vi "Compute Max Level.vi"(0 "File in":refnum<class "File.lvclass">, 1 "Filter in":refnum<class "Filter.lvclass">, 5 "Level in":refnum<class "Level.lvclass">, 7 "Fs (Hz)":dbl, 9 "Vmax":dbl, 11 "error in (no error)":errorcluster) -> (4 "File out":refnum<class "File.lvclass">, 6 "Level thru":refnum<class "Level.lvclass">, 10 "Lmax":dbl, 15 "error out":errorcluster)   [LabVIEW 2020, in "File.lvclass"]
uses:
  File.lvclass
  Level/Level.lvclass
  Filter/Filter.lvclass
  Level/Level.lvclass/Level.ctl
  File.lvclass/File.ctl
  aa2963da-88b9-45dc-ab26-109d9a687043.vi
  6b23c93a-1c02-4248-999f-575423126d1e.vi
  439032d3-8d6b-4fc5-a9ed-bfbf51eac51d.vi
  e43c2267-94e9-47ec-9fe9-8526f4fbc379.vi
  Level/Read Units.vi
  Utility VIs/Math VIs/FFT x(t) to dB,Degrees (1D).vi
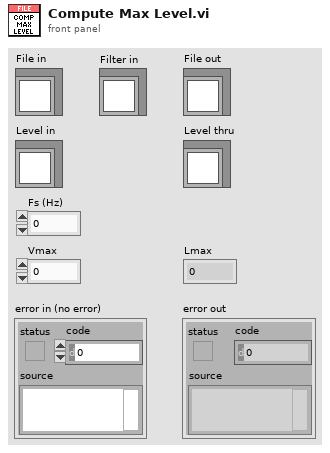
[diagram p1: front panel]
types:
  T1 = typedef "Level.lvclass/LevelUnits.ctl" = enum16{"dB atten", "dB SPL", "dB Vrms", "Volts", "dB mW", "mW", "dB HL", "dB SL"}
  T2 = cluster{"Freq (Hz)":dbl[], "Mag (dB SPL)":dbl[], "Phase (deg)":dbl[]}
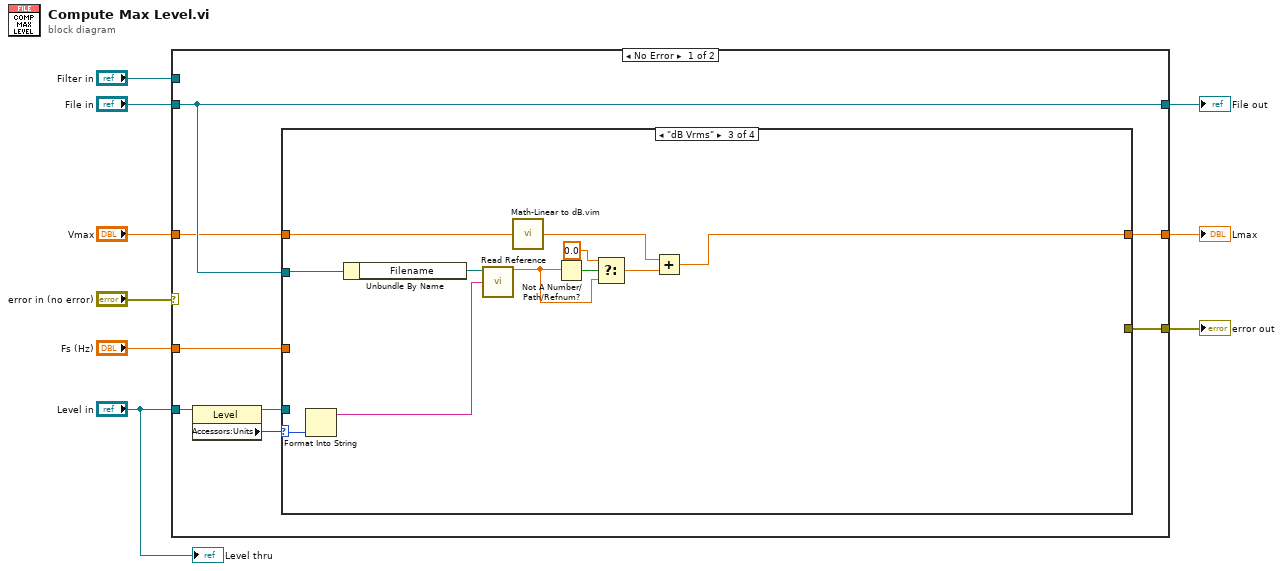
[diagram p0: block diagram]
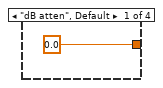
[diagram p2: hidden frame]
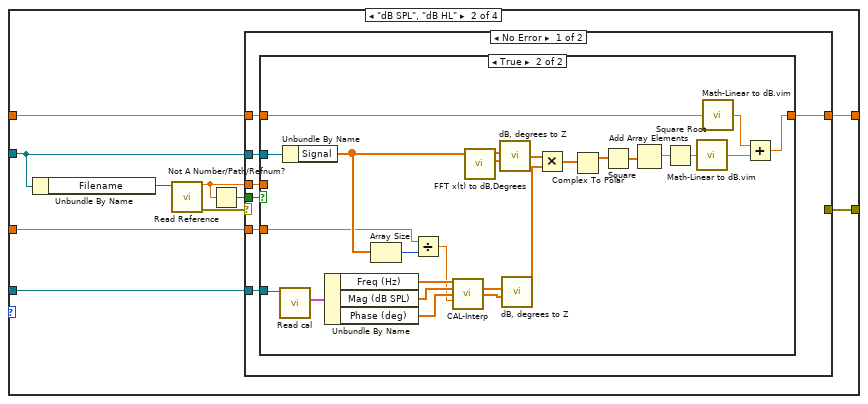
[diagram p3: hidden frame]
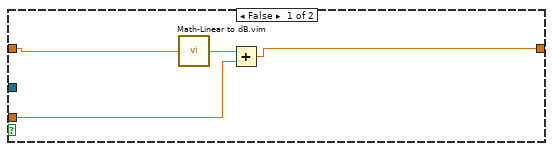
[diagram p4: hidden frame]
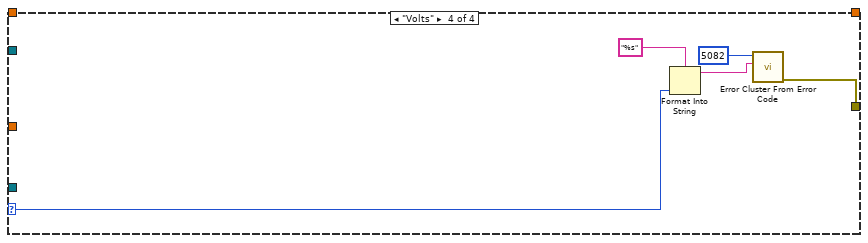
[diagram p6: hidden frame]
diagram:
  n1 = case shown="No Error" "error in (no error)" {
    selector: "error in (no error)" -> [_ w82]
    tunnel: "Filter in" -> [_ _]
    tunnel: [w14 w83] -> w6
    tunnel: "File in" -> [w14 w83]
    tunnel: "Level in" -> [w16 _]
    tunnel: [w15 _] -> w5
    tunnel: [w13 w82] -> w4
    tunnel: "Vmax" -> [w12 _]
    tunnel: "Fs (Hz)" -> [w10 _]
    frame No Error {
      n2 = property class="Level"(reference=w16) -> (reference out=w11:refnum<class "Level.lvclass">, "Accessors:Units"=w17:T1)  [unwired: 1 in, 1 out]
      n3 = case shown="\"dB Vrms\"" w17 {
        selector: w17 -> [_ _ w73 w77]
        tunnel: [0.0 ("Reference Level") w28 w66 _] -> w15
        tunnel: [_ w27 _ w78] -> w13
        tunnel: w14 -> [_ w26 w74 _]
        tunnel: w12 -> [_ w21 w76 _]
        tunnel: w11 -> [_ w20 _ _]
        tunnel: w10 -> [_ w19 _ _]
        frame "dB atten", Default {
        }
        frame "dB SPL", "dB HL" {
          n4 = Unbundle By Name(w26) -> ("Filename"=w22:path)
          n5 = call "Read Reference.vi"("Wave File"=w22) -> ("Reference (dB)"=w23:dbl, "error out"=w25:errorcluster)  [unwired: 12 in, 1 out]
          n6 = Not A Number/Path/Refnum?(number/path/refnum=w23) -> (NaN/Path/Refnum?=w24:bool)
          n7 = case shown="No Error" w25 {
            selector: w25 -> [_ w65]
            tunnel: [w35 _] -> w28
            tunnel: [_ w65] -> w27
            tunnel: w26 -> [w34 _]
            tunnel: w24 -> [w33 _]
            tunnel: w23 -> [w32 _]
            tunnel: w21 -> [w31 _]
            tunnel: w20 -> [w30 _]
            tunnel: w19 -> [w29 _]
            frame No Error {
              n8 = case shown="True" w33 {
                tunnel: [w37 w47] -> w35
                tunnel: w34 -> [_ w64]
                tunnel: w32 -> [w38 _]
                tunnel: w31 -> [w36 w50]
                tunnel: w30 -> [_ w49]
                tunnel: w29 -> [_ w40]
                frame False {
                  n9 = call "Math-Linear to dB.vim"("linear"=w36) -> ("dB"=w39:dbl)
                  n10 = Add(x=w39, y=w38) -> (x+y=w37:dbl)
                }
                frame True {
                  n11 = call "Read cal.vi"("Level in"=w49) -> ("cal"=w48:T2)  [unwired: 8 in, 2 out]
                  n12 = Unbundle By Name(w64) -> ("Signal"=w42:dbl[])
                  n13 = Unbundle By Name(w48) -> ("Freq (Hz)"=w46:dbl[], "Mag (dB SPL)"=w45:dbl[], "Phase (deg)"=w44:dbl[])
                  n14 = Array Size(array=w42) -> (size(s)=w43:i32)
                  n15 = Divide(x=w40, y=w43) -> (x/y=w41:dbl)
                  n16 = call "CAL-Interp.vi"("Frequency (Hz)"=w46, "Magnitude (dB)"=w45, "Phase (degrees)"=w44, "df (Hz)"=w41) -> ("Interp Magnitude (dB)"=w53:dbl[], "Interp Phase (degrees)"=w54:dbl[])  [unwired: 8 in, 2 out]
                  n17 = call-poly "FFT x(t) to dB,Degrees.vi"("X"=w42) -> ("+Freq Phase of FFT (degrees)"=w56:dbl[], "+Freq. Mag of FFT (dB rms)"=w55:dbl[])  [unwired: 8 in, 1 out]
                  n18 = call "dB, degrees to Z.vi"("Magnitude (dB)"=w55, "Phase (degrees)"=w56) -> ("Z"=w62:cdb[])  [unwired: 5 in]
                  n19 = call "dB, degrees to Z.vi"("Magnitude (dB)"=w53, "Phase (degrees)"=w54) -> ("Z"=w52:cdb[])  [unwired: 5 in]
                  n20 = Multiply(x=w62, y=w52) -> (x*y=w63:cdb[])
                  n21 = Complex To Polar(r * e^(i*theta)=w63) -> (r=w60:dbl[])  [unwired: 1 out]
                  n22 = Square(x=w60) -> (x^2=w57:dbl[])
                  n23 = Add Array Elements(numeric array=w57) -> (sum=w58:dbl)
                  n24 = Square Root(x=w58) -> (sqrt(x)=w59:dbl)
                  n25 = call "Math-Linear to dB.vim"("linear"=w59) -> ("dB"=w61:dbl)
                  n26 = call "Math-Linear to dB.vim"("linear"=w50) -> ("dB"=w51:dbl)
                  n27 = Add(x=w51, y=w61) -> (x+y=w47:dbl)
                }
              }
            }
            frame Error {
            }
          }
        }
        frame "dB Vrms" {
          n28 = Format Into String(w73) -> (resulting string=w72:string)  [unwired: 3 in, 1 out]
          n29 = Unbundle By Name(w74) -> ("Filename"=w75:path)
          n30 = call "Read Reference.vi"("Wave File"=w75, "refUnits"=w72) -> ("Reference (dB)"=w70:dbl)  [unwired: 11 in, 2 out]
          n31 = call "Math-Linear to dB.vim"("linear"=w76) -> ("dB"=w67:dbl)
          n32 = Not A Number/Path/Refnum?(number/path/refnum=w70) -> (NaN/Path/Refnum?=w71:bool)
          n33 = Select(t=0.0, s=w71, f=w70) -> (s? t:f=w68:dbl)
          n34 = Add(x=w67, y=w68) -> (x+y=w66:dbl)
        }
        frame "Volts" {
          n35 = Format Into String(format string="%s", w77) -> (resulting string=w80:string)  [unwired: 2 in, 1 out]
          n36 = call <vilib>:"Error Cluster From Error Code.vi"("error message (\"\")"=w80, "error code (0)"=5082) -> ("error out"=w78:errorcluster)  [unwired: 7 in]
        }
      }
    }
    frame Error {
    }
  }
  "error out" <- w4
  "File out" <- w6
  "Lmax" <- w5
  "Level thru" <- "Level in"
